vi "LabView.vi"() -> ()   [LabVIEW 2024]
panel:
  out "Weight":dbl(knob) scale=0.0..7.0 scale format="%1.3f"
  out "Offset, V":dbl format="%01.3f"
  out "Vdiff, mv":dbl format="%01.3f"
  in  "stop":bool
  in  "Tare":bool
  out "SCC, V":dbl(knob) scale=0.0..5.0 scale format="%1.3g"
  out "AtoDOut":i16 format="%04x"
  in  "COMM_in":refnum<visa-resource-name>
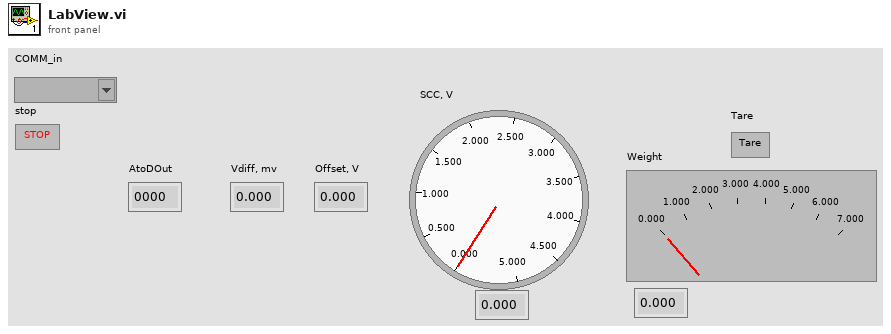
[diagram p1: front panel]
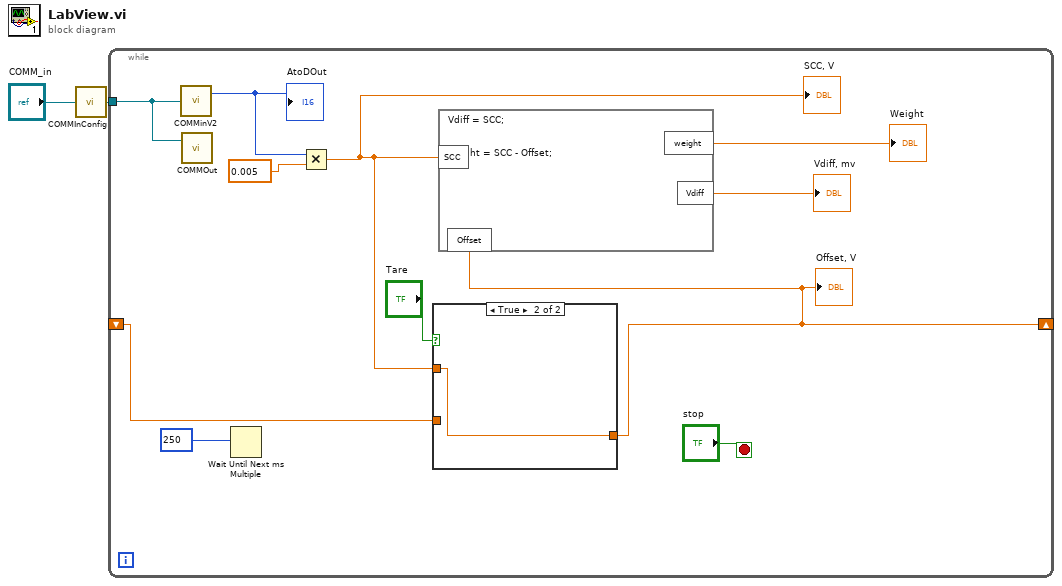
[diagram p0: block diagram]
diagram:
  n1 = call "COMMInConfig.vi"("COMM_in"="COMM_in") -> ("COMM_Name"=w1:refnum<visa-resource-name>)
  n2 = while {
    tunnel: w1 -> [w13]
    shift-right: [w4] -> _
    shift-left: _ -> [w7]
    stop <- "stop" stop-if-true
    n3 = call "COMMinV2.vi"("VISA resource name"=w13) -> ("AtoDOut"=w11:i16)  [unwired: 1 out]
    "AtoDOut" <- w11
    n4 = call "COMMOut.vi"("VISA resource name"=w13) -> ()  [unwired: 1 in]
    n5 = Wait Until Next ms Multiple(millisecond multiple=250) -> ()  [unwired: 1 out]
    n6 = Multiply(x=w11, y=0.005) -> (x*y=w6:dbl)
    "SCC, V" <- w6
    n7 = case shown="True" "Tare" {
      tunnel: w7 -> [w14 _]
      tunnel: [w14 w15] -> w4
      tunnel: w6 -> [_ w15]
      frame False {
      }
      frame True {
      }
    }
    "Offset, V" <- w4
    n8 = formula code="Vdiff = SCC;\n\n\nweight = SCC - Offset;"("SCC"=w6, "Offset"=w4) -> ("Vdiff"=→"Vdiff, mv":dbl, "weight"=→"Weight":dbl)
  }
